vi "Write Class Tree.vi"(8 "error in (no error)":errorcluster, 10 "Class Tree Reference":refnum<vi>, 11 "Tag Tree In":refnum<class "LVCLass Tree.lvclass">) -> (0 "error out":errorcluster, 3 "Tag Tree Out":refnum<class "LVCLass Tree.lvclass">)   [LabVIEW 2020, in "Tree Helpers.lvlib" / "LVCLass Tree.lvclass"]
uses:
  LVCLass Tree.lvclass
  LVCLass Tree.lvclass/LVCLass Tree.ctl
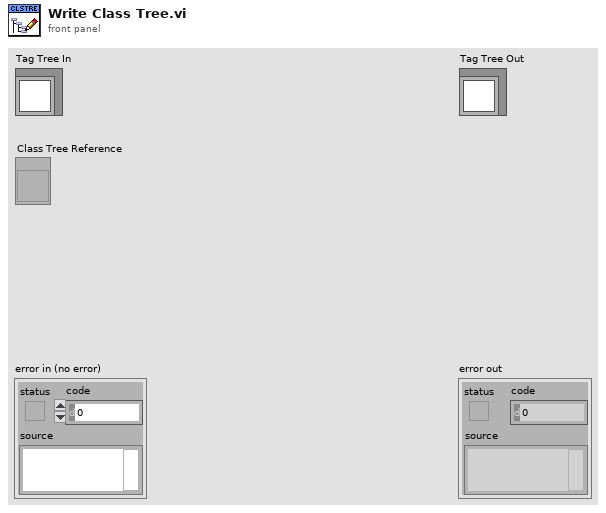
[diagram p1: front panel]
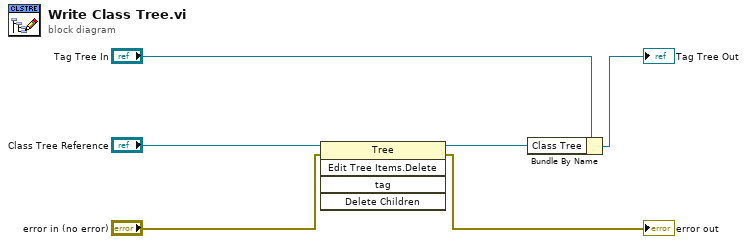
[diagram p0: block diagram]
diagram:
  n1 = invoke class="Tree" method="Edit Tree Items.Delete"(reference="Class Tree Reference", error in="error in (no error)") -> (reference out=w3:refnum<vi>, error out=→"error out":errorcluster)  [unwired: 3 in, 3 out]
  n2 = Bundle By Name(cluster="Tag Tree In", "Class Tree"=w3) -> (→"Tag Tree Out":refnum<class "LVCLass Tree.lvclass">)
